vi "RP set frequency.vi"(8 "Error In":errorcluster, 10 "Frequency":dbl, 11 "connection ID":refnum<k5>) -> (0 "Error Out":errorcluster, 2 "Phase increment":u64=1717987, 3 "connection ID out":refnum<k5>)   [LabVIEW 2015]
uses:
  RP Command.ctl
panel:
  out "x*y":dbl
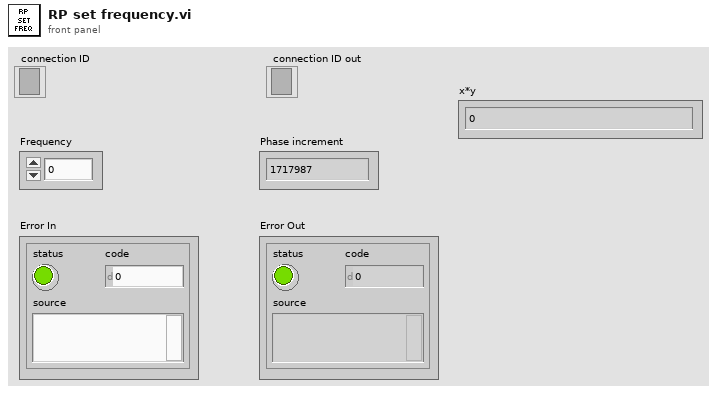
[diagram p1: front panel]
types:
  T1 = typedef "RP Command.ctl" = enum16{"Set frequency", "Arm and get data", "Stop server", "Get status", "Get temperature", "Set decimation", "Arm", "Software trigger", "Get whole buffer", "Get chunk", "System call", "Get config", "Set config", "Read FIFO", "Play pattern", "Set frequency batch"}
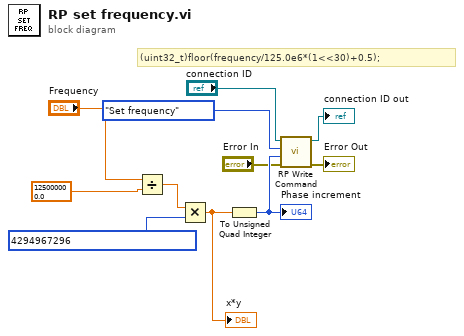
[diagram p0: block diagram]
diagram:
  # "(uint32_t)floor(frequency/125.0e6*(1<<30)+0.5);"
  n1 = Divide(x="Frequency", y=125000000.0) -> (x/y=w9:dbl)
  n2 = Multiply(x=w9, y=i64 4294967296) -> (x*y=w8:dbl)
  "x*y" <- w8
  n3 = To Unsigned Quad Integer(1:w8) -> (0:w5:u64)
  "Phase increment" <- w5
  n4 = call "RP Write Command.vi"("Error In"="Error In", "Command payload"=w5, "Command number"=RP_Command."Set frequency", "connection ID"="connection ID") -> ("Error Out"=→"Error Out":errorcluster, "connection ID out"=→"connection ID out":refnum<k5>)  [unwired: 5 in, 1 out]
